vi "Кодер манчестера (SubVI).vi"(10 "Вход":bool[](array[boolean])) -> (2 "Выход":bool[](array[boolean]))   [LabVIEW 2015]
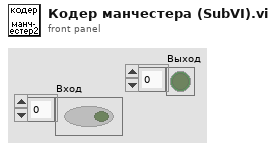
[diagram p1: front panel]
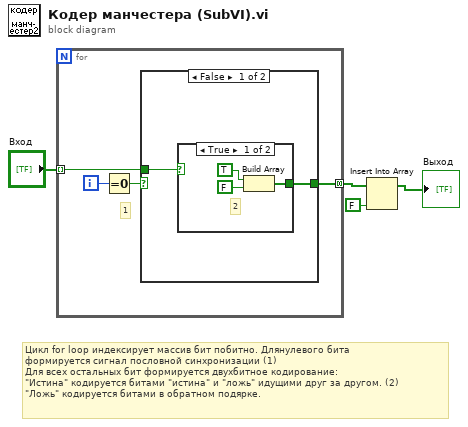
[diagram p0: block diagram]
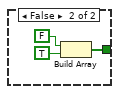
[diagram p2: hidden frame]
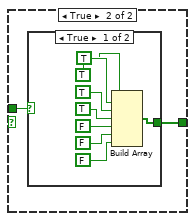
[diagram p3: hidden frame]
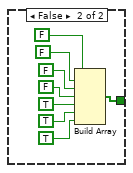
[diagram p4: hidden frame]
diagram:
  # "Цикл for loop индексирует массив бит побитно. Длянулевого бита \nформируется сигнал пословной синхронизации (1)\nДля всех остальных бит формируется двухбитное кодирование:\n\"Истина\" кодируется битами \"истина\" и \"ложь\" идущими друг за другом. (2)\n\"Ложь\" кодируется битами в обратном подярке."
  n1 = for {
    tunnel: "Вход" -> [w8] mode=indexing
    tunnel: [w7] -> w3 mode=concatenating
    i -> [w6]
    # "1"
    n2 = Equal To 0?(x=w6) -> (x = 0?=w5:bool)
    n3 = case shown="False" w5 {
      tunnel: w8 -> [w10 w17]
      tunnel: [w9 w18] -> w7
      frame False {
        n4 = case shown="True" w10 {
          tunnel: [w11 w14] -> w9
          frame True {
            # "2"
            n5 = Build Array(TRUE, FALSE) -> (w11:bool[])
          }
          frame False {
            n6 = Build Array(FALSE, TRUE) -> (w14:bool[])
          }
        }
      }
      frame True {
        n7 = case shown="True" w17 {
          tunnel: [w20 w28] -> w18
          frame True {
            n8 = Build Array(TRUE, TRUE, TRUE, TRUE, FALSE, FALSE, FALSE) -> (w20:bool[])
          }
          frame False {
            n9 = Build Array(FALSE, FALSE, FALSE, FALSE, TRUE, TRUE, TRUE) -> (w28:bool[])
          }
        }
      }
    }
  }
  n10 = Insert Into Array(array=w3, new element=FALSE ("new element/subarray")) -> (→"Выход":bool[])  [unwired: 1 in]
